vi "write_read_ic6.vi"(1 "Input string":string) -> (0 "Output string":string)   [LabVIEW 2012]
panel:
  out "error out":errorcluster {"code" format="%x"}
  in  "error in (no error)":errorcluster {"code" format="%x"}
  in  "Read delay (ms)":u32=50
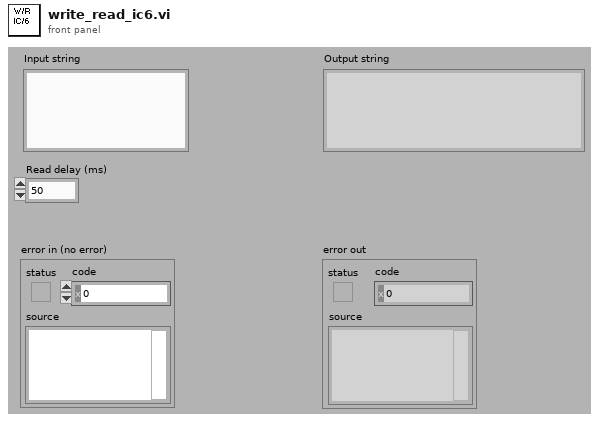
[diagram p1: front panel]
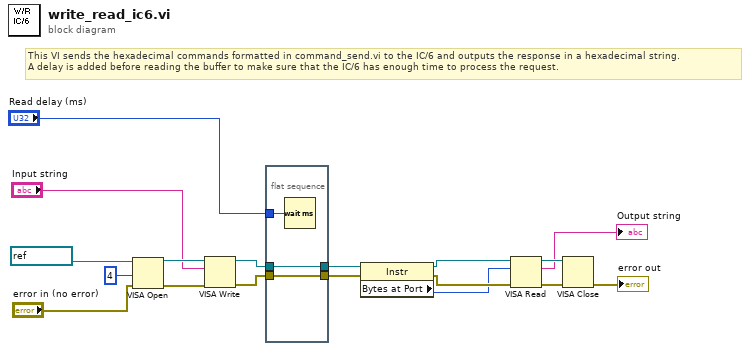
[diagram p0: block diagram]
diagram:
  # "This VI sends the hexadecimal commands formatted in command_send.vi to the IC/6 and outputs the response in a hexadecimal string.\nA delay is added before reading the buffer to make sure that the IC/6 has enough time to process the request."
  n1 = VISA Open(access mode=u32 4, error in (no error)="error in (no error)", VISA resource name=refnum<visa-resource-name> "COM1" ("IC/6 object")) -> (VISA resource name=w13:refnum<visa-resource-name>, error out=w12:errorcluster)  [unwired: 2 in]
  n2 = VISA Write(VISA resource name=w13, write buffer="Input string", error in (no error)=w12) -> (VISA resource name out=w11:refnum<visa-resource-name>, error out=w10:errorcluster)  [unwired: 1 out]
  n3 = flat-sequence {
    tunnel: w11 -> [w20]
    tunnel: w10 -> [w19]
    tunnel: "Read delay (ms)" -> [w21]
    tunnel: [w20] -> w6
    tunnel: [w19] -> w5
    frame #0 {
      n4 = Wait (ms)(milliseconds to wait=w21) -> ()  [unwired: 1 out]
    }
  }
  n5 = property class="Instr"(reference=w6, error in=w5) -> (reference out=w4:refnum<visa-resource-name>, error out=w7:errorcluster, "Bytes at Port"=w3:u32)
  n6 = VISA Read(VISA resource name=w4, byte count=w3, error in (no error)=w7) -> (VISA resource name out=w14:refnum<visa-resource-name>, read buffer=→"Output string":string, error out=w15:errorcluster)  [unwired: 1 out]
  n7 = VISA Close(VISA resource name=w14, error in (no error)=w15) -> (error out=→"error out":errorcluster)
